vi "Soln.vi"(1 "Num2":dbl, 2 "Num1":dbl) -> (0 "Sum":dbl)   [LabVIEW 2015]
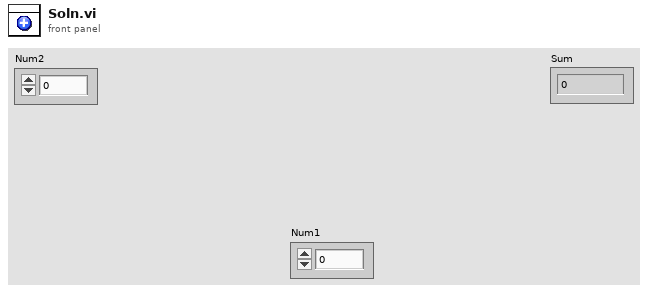
[diagram p1: front panel]
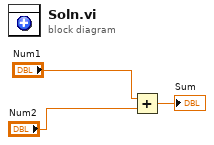
[diagram p0: block diagram]
diagram:
  n1 = Add(x="Num1", y="Num2") -> (x+y=→"Sum":dbl)
